vi "EnableDisableRow.vi"(6 "Cell Position":T1, 7 "Disable / Enable":bool caption="Enable?", 8 "error in (no error)":errorcluster, 9 "Table CtlRef In":refnum<vi>, 10 "Table Data in":string[][](array[string]), 11 "Col Array in":refnum<class "Column.lvclass">[](array[class])) -> (0 "error out":errorcluster, 1 "Table CtlRef Out":refnum<vi>, 2 "Table Data out":string[][](array[string]))   [LabVIEW 2013]
uses:
  <vilib>/Utility/miscctls.llb/LVRowAndColumnTypeDef.ctl
  ColumnVIs/Column/Column.lvclass
  Globals/DisabledColorGlobal.vi
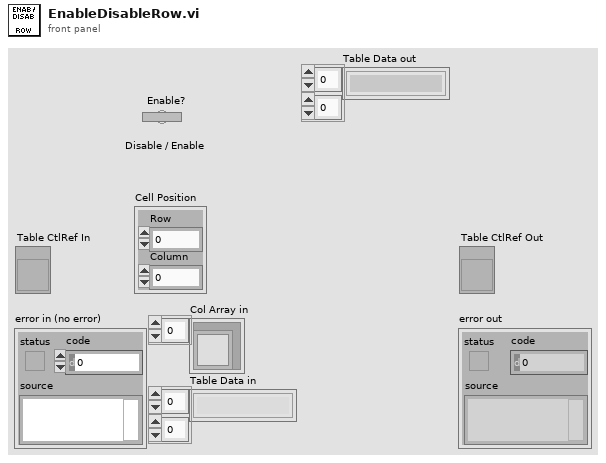
[diagram p1: front panel]
types:
  T1 = typedef "LVRowAndColumnTypeDef.ctl" = cluster{"Row":i32, "Column":i32}
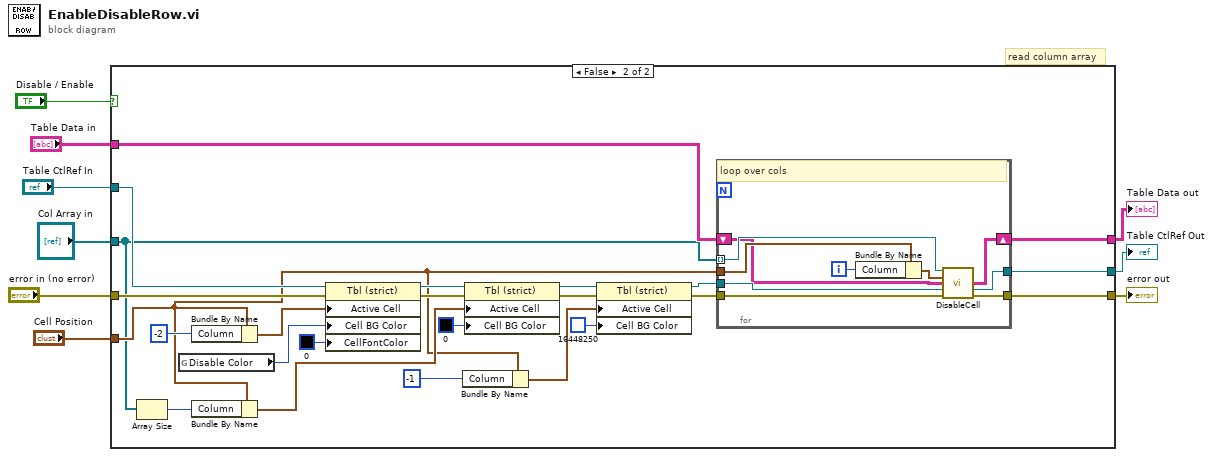
[diagram p0: block diagram]
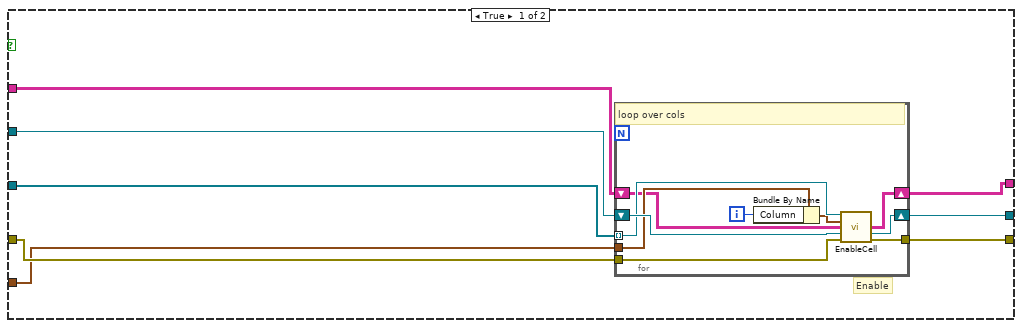
[diagram p2: hidden frame]
diagram:
  # "read column array"
  n1 = case shown="False" "Disable / Enable" {
    tunnel: "Col Array in" -> [w17 w33]
    tunnel: "error in (no error)" -> [w16 w46]
    tunnel: [w15 w51] -> w9
    tunnel: [w14 w50] -> w8
    tunnel: "Table CtlRef In" -> [w13 w47]
    tunnel: "Cell Position" -> [w12 w35]
    tunnel: "Table Data in" -> [w11 w49]
    tunnel: [w10 w48] -> w1
    frame True {
      # "Enable"
      n2 = for {
        tunnel: [w27] -> w15
        tunnel: w16 -> [w24]
        tunnel: w17 -> [w23] mode=indexing
        tunnel: w12 -> [w20]
        shift-right: [w26] -> w14
        shift-left: w13 -> [w25]
        shift-right: [w18] -> w10
        shift-left: w11 -> [w19]
        i -> [w22]
        # "loop over cols"
        n3 = Bundle By Name(cluster=w20, "Column"=w22) -> (w21:T1)
        n4 = call-dynamic "EnableCell.vi"("Column in"=w23, "Cell Position"=w21, "Table Data in"=w19, "Table CtlRef In"=w25, "error in (no error)"=w24) -> ("Table Data out"=w18:string[][], "Table CtlRef Out"=w26:refnum<vi>, "error out"=w27:errorcluster)  [unwired: 7 in, 1 out]
      }
    }
    frame False {
      n5 = Array Size(array=w33) -> (size(s)=w32:i32)
      n6 = global read "DisabledColorGlobal.vi" "Disable Color"() -> (w44:u32)
      n7 = Bundle By Name(cluster=w35, "Column"=-2) -> (w37:T1)
      n8 = Bundle By Name(cluster=w35, "Column"=w32) -> (w36:T1)
      n9 = property class="Tbl (strict)"(reference=w47, error in=w46, "Active Cell"=w37, "Cell BG Color"=w44, "CellFontColor"=u32 0 ("Color Box")) -> (reference out=w41:refnum<vi>, error out=w40:errorcluster)
      n10 = Bundle By Name(cluster=w35, "Column"=-1) -> (w34:T1)
      n11 = property class="Tbl (strict)"(reference=w41, error in=w40, "Active Cell"=w36, "Cell BG Color"=u32 0 ("Color Box")) -> (reference out=w43:refnum<vi>, error out=w42:errorcluster)
      n12 = property class="Tbl (strict)"(reference=w43, error in=w42, "Active Cell"=w34, "Cell BG Color"=u32 16448250 ("Color Box")) -> (reference out=w38:refnum<vi>, error out=w39:errorcluster)
      n13 = for {
        tunnel: [w61] -> w51
        tunnel: [w60] -> w50
        tunnel: w38 -> [w59]
        tunnel: w39 -> [w58]
        tunnel: w33 -> [w57] mode=indexing
        tunnel: w35 -> [w54]
        shift-right: [w52] -> w48
        shift-left: w49 -> [w53]
        i -> [w56]
        # "loop over cols"
        n14 = Bundle By Name(cluster=w54, "Column"=w56) -> (w55:T1)
        n15 = call-dynamic "DisableCell.vi"("Column in"=w57, "Cell Position"=w55, "Table Data in"=w53, "Table CtlRef In"=w59, "error in (no error)"=w58) -> ("Table Data out"=w52:string[][], "Table CtlRef Out"=w60:refnum<vi>, "error out"=w61:errorcluster)  [unwired: 7 in, 1 out]
      }
    }
  }
  "error out" <- w9
  "Table CtlRef Out" <- w8
  "Table Data out" <- w1
